vi "delete_element.vi"   [LabVIEW 2016]
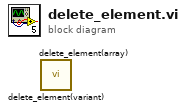
[diagram p0: block diagram]
diagram:
  n1 = call "delete_element(variant).vi"() -> ()  [unwired: 9 in, 3 out]
  n2 = call "delete_element(array).vi"() -> ()  [unwired: 8 in, 4 out]
